vi "Image To Tensor.vi"(8 "error in (no error)":errorcluster, 11 "image data IN":T1) -> (0 "error out":errorcluster, 2 "Data":sgl[](array[numeric]))   [LabVIEW 2017, in "process_EfficientNet_B4.lvlib"]
doc: "Created IvanLis by LabVIEW Portal\nProfile: http://labviewportal.org/memberlist.php?mode=viewprofile&u=987\neMail: IvanLisanov@gMail.com\nTelegram: https://t.me/IvanLis"
uses:
  process_EfficientNet_B4.lvlib
  image_vi/image.lvlib
  <vilib>/picture/picture.llb/imagedata.ctl
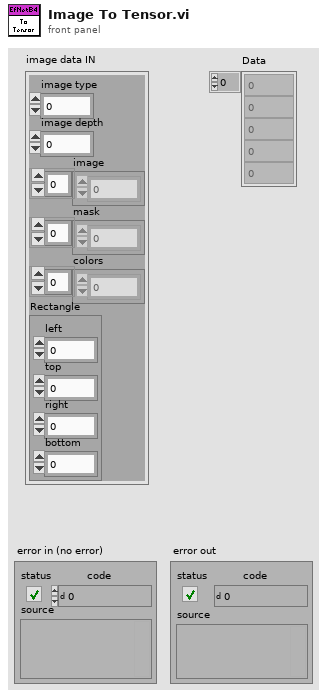
[diagram p1: front panel]
types:
  T1 = typedef "imagedata.ctl" = cluster{"image type":i32, "image depth":i32, "image":u8[], "mask":u8[], "colors":u32[], "Rectangle":cluster{"left":i16, "top":i16, "right":i16, "bottom":i16}}
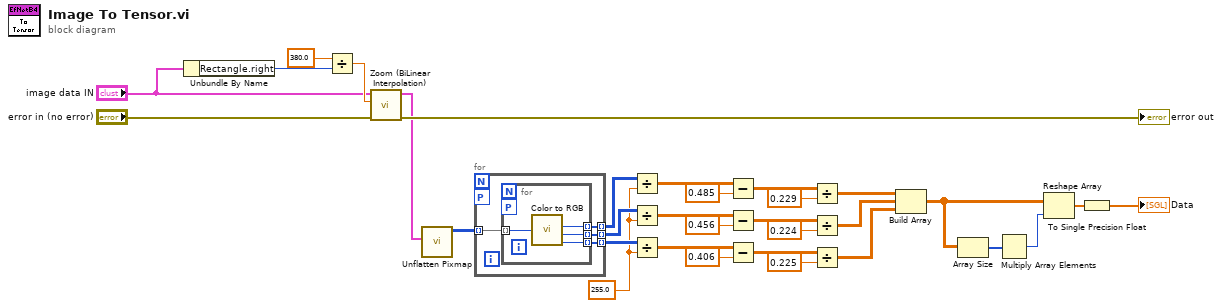
[diagram p0: block diagram]
diagram:
  w20 = 255.0 ("y")
  n1 = Unbundle By Name("image data IN") -> ("Rectangle.right"=w30:i16)
  n2 = Divide(x=380.0, y=w30) -> (x/y=w32:dbl)
  n3 = call "Zoom (BiLinear Interpolation).vi"("error IN"="error in (no error)", "Zoom Coefficient"=w32, "image data IN"="image data IN") -> ("error OUT"=→"error out":errorcluster, "image data OUT"=w19:T1)  [unwired: 7 in]
  n4 = call <vilib>:"Unflatten Pixmap.vi"("image data"=w19) -> ("24-bit pixmap"=w28:u32[][])  [unwired: 10 out]
  n5 = for {
    tunnel: w28 -> [w36] mode=indexing
    tunnel: [w35] -> w21 mode=indexing
    tunnel: [w34] -> w22 mode=indexing
    tunnel: [w33] -> w23 mode=indexing
    workers-P: _ -> [_]
    n6 = for {
      tunnel: w36 -> [w37] mode=indexing
      tunnel: [w40] -> w35 mode=indexing
      tunnel: [w39] -> w34 mode=indexing
      tunnel: [w38] -> w33 mode=indexing
      workers-P: _ -> [_]
      n7 = call <vilib>:"Color to RGB.vi"("Color"=w37) -> ("R"=w40:u8, "G"=w39:u8, "B"=w38:u8)  [unwired: 1 out]
    }
  }
  n8 = Divide(x=w21, y=w20) -> (x/y=w18:dbl[][])
  n9 = Divide(x=w22, y=w20) -> (x/y=w7:dbl[][])
  n10 = Divide(x=w23, y=w20) -> (x/y=w5:dbl[][])
  n11 = Subtract(x=w18, y=0.485) -> (x-y=w16:dbl[][])
  n12 = Subtract(x=w7, y=0.456) -> (x-y=w8:dbl[][])
  n13 = Subtract(x=w5, y=0.406) -> (x-y=w10:dbl[][])
  n14 = Divide(x=w16, y=0.229) -> (x/y=w15:dbl[][])
  n15 = Divide(x=w8, y=0.224) -> (x/y=w6:dbl[][])
  n16 = Divide(x=w10, y=0.225) -> (x/y=w4:dbl[][])
  n17 = Build Array(w15, w6, w4) -> (w25:dbl[][][])
  n18 = Array Size(array=w25) -> (size(s)=w24:i32[])
  n19 = Multiply Array Elements(1:w24) -> (0:w26:i32)
  n20 = Reshape Array(w25, w26) -> (w27:dbl[])
  n21 = To Single Precision Float(number=w27) -> (single precision float=→"Data":sgl[])
